vi "Vision Research Phantom Series PhGetCameraTime.vi"(0 "CN in":u32=1, 5 "Error In (no error)":errorcluster) -> (14 "CN out":u32=1, 15 "pTime64":T1 {"fractions" format="%32.0f"}, 19 "Error Out":errorcluster)   [LabVIEW 2013, in "VRI.lvlib"]
doc: "PhCon.dll\n\nPhGetCameraTime\nHRESULT PhGetCameraTime(UINT CN, PTIME64 pTime64);\n\nParameters Description\nCN (in) Camera number.\npTime (out) The current time in the TIME64 format.\nReturn HRESULT (0=Ok)\nComments Read the camera clock. The fractions of second\n are important for the information in the bit 0 \n and 1: the presence of IRIG synchronization \n signal and the Event binary input. Use the\n standard ctime function to convert it to a \n string of characters.\n\nWritten by:\nBLOOMY CONTROLS, INC\nWINDSOR, CT 06095, USA\n860-298-9925\nwww.bloomy.com\nV1.0.0\nMay, 2004"
uses:
  VRI.lvlib
  _Type Defs/PHCon Time64.ctl
  Phantom DLLs/PhCon.Dll
panel:
  # "For instructions on the use of this VI, press Ctrl+H to display the help window and move the mouse over the icon, controls, and indicators"
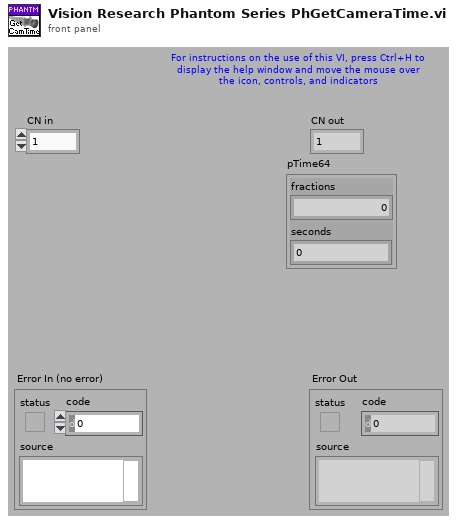
[diagram p1: front panel]
types:
  T1 = typedef "VRI.lvlib/PHCon Time64.ctl" = cluster{"fractions":u32, "seconds":u32}
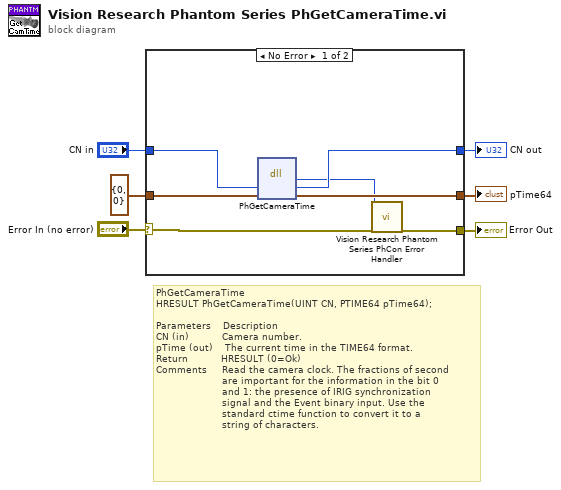
[diagram p0: block diagram]
diagram:
  # "PhGetCameraTime\nHRESULT PhGetCameraTime(UINT CN, PTIME64 pTime64);\n\nParameters    Description\nCN (in)           Camera number.\npTime (out)    The current time in the TIME64 format.\nReturn           HRESULT (0=Ok)\nComments     Read the camera clock. The fractions of second\n                      are important for the information in the bit 0 \n                      and 1: the presence of IRIG synchronization \n                      signal and the Event binary input. Use the\n                      standard ctime function to convert it to a \n                      string of characters."
  n1 = case shown="No Error" "Error In (no error)" {
    selector: "Error In (no error)" -> [w13 w16]
    tunnel: [w12 w16] -> w5
    tunnel: "CN in" -> [w11 w15]
    tunnel: [w10 w15] -> w3
    tunnel: T1 {"fractions"=0, "seconds"=0} ("Time64") -> [w9 w14]
    tunnel: [w8 w14] -> w1
    frame No Error {
      n2 = dll-call lib="C:/Projects/SDK/64-bit/Vision Research Phantom Series Labview Driver/Phantom DLLs/PhCon.dll" fn="PhGetCameraTime"("CN"=w11, "Time64"=w9) -> ("HRESULT"=w7:i32, "CN"=w10:u32, "Time64"=w8:T1)  [unwired: 3 in, 2 out]
      n3 = call "Vision Research Phantom Series PhCon Error Handler.vi"("ErrNo"=w7, "Error In (no error)"=w13) -> ("Error Out"=w12:errorcluster)  [unwired: 17 out]
    }
    frame Error {
    }
  }
  "Error Out" <- w5
  "CN out" <- w3
  "pTime64" <- w1
